vi "Sine.Generate.vi"(11 "Settings":T1={"Amplitude"=0.0, "Offset"=0.0, "Periods/Tick"=0.0002500000409781933}) -> (3 "Output":fxp<+/-,48,9>)   [LabVIEW 2015, in "Speciality FPGA IO.lvlib"]
uses:
  Speciality FPGA IO.lvlib
  Types/Sine.Generate.Settings.ctl
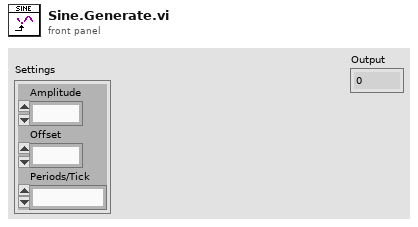
[diagram p1: front panel]
types:
  T1 = typedef "Speciality FPGA IO.lvlib/Sine.Generate.Settings.ctl" = cluster{"Amplitude":fxp<+/-,32,8>, "Offset":fxp<+/-,32,8>, "Periods/Tick":fxp<+,32,0>}
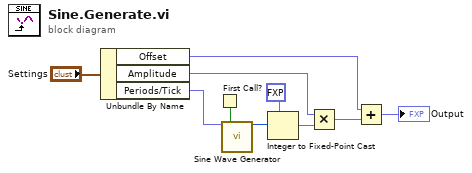
[diagram p0: block diagram]
diagram:
  n1 = Unbundle By Name("Settings") -> ("Offset"=w2:fxp<+/-,32,8>, "Amplitude"=w3:fxp<+/-,32,8>, "Periods/Tick"=w1:fxp<+,32,0>)
  n2 = First Call?() -> (First Call?: T/F=w10:bool)
  n3 = call "Sine Wave Generator"("frequency (periods/tick)"=w1, "reset"=w10) -> ("sine out"=w8:i16)  [unwired: 13 in]
  n4 = Integer to Fixed-Point Cast(fixed-point type=fxp<+/-,16,1> 0.0, integer=w8) -> (fixed-point=w6:fxp<+/-,16,1>)
  n5 = Multiply(x=w3, y=w6) -> (x*y=w9:fxp<+/-,48,9>)
  n6 = Add(x=w2, y=w9) -> (x+y=→"Output":fxp<+/-,48,9>)
